vi "TestGEA2.vi"() -> ()   [LabVIEW 2009]
panel:
  out "Array 2":errorcluster[](array[cluster])
  out "Array":i32[](array[numeric])
  out "GetPendingMessage_Out":T1 {"pu8DataBufferToFill_Out" format="%.0x"}
  in  "error in (no error)":errorcluster
  in  "Data_To_Send":T2={"pu8BufferToSend"=[255, 86], "u8TargetAddress"=96} {"u8TargetAddress" format="%.0x"}
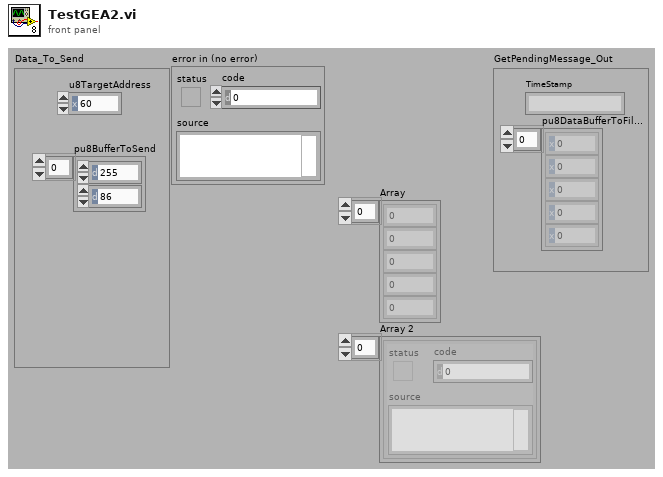
[diagram p1: front panel]
types:
  T1 = cluster{"TimeStamp":string, "pu8DataBufferToFill_Out":u8[]}
  T2 = cluster{"pu8BufferToSend":u8[], "u8TargetAddress":u8}
  T3 = enum16{"GEA_Connect", "GEA_Disconnect", "GEA_GetPendingMessages", "GEA_SendMessage"}[]
  T4 = cluster{"Com Port":i32, "Speed":i32, "MyAddress":u8}
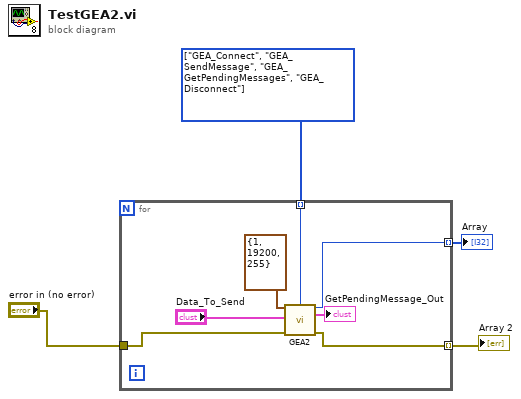
[diagram p0: block diagram]
diagram:
  w4 = T3 [enum."GEA_Connect", enum."GEA_SendMessage", enum."GEA_GetPendingMessages", enum."GEA_Disconnect"] items=["GEA_Connect", "GEA_Disconnect", "GEA_GetPendingMessages", "GEA_SendMessage"]
  n1 = for {
    tunnel: w4 -> [w11] mode=indexing
    tunnel: [w5] -> w1 mode=indexing
    tunnel: "error in (no error)" -> [w8]
    tunnel: [w7] -> w2 mode=indexing
    n2 = call "GEA2.vi"("Connect Data"=T4 {"Com Port"=1, "Speed"=19200, "MyAddress"=255}, "Enum"=w11, "Data_To_Send"="Data_To_Send", "error in (no error)"=w8) -> ("return type"=w5:i32, "GetPendingMessage_Out"=→"GetPendingMessage_Out":T1, "error out"=w7:errorcluster)  [unwired: 9 in]
  }
  "Array" <- w1
  "Array 2" <- w2
